vi "CreatePublicEvents.vi"(8 "error in (no error)":errorcluster, 11 "Control Experiment":refnum<class "SMO.Control Experiment.lvclass">) -> (0 "error out":errorcluster, 3 "Control Experiment out":refnum<class "SMO.Control Experiment.lvclass">)   [LabVIEW 2019, in "SMO.Control Experiment.lvclass"]
doc: "---------------------------------------------------------------\nJKI State Machine Objects™\nhttp://jki.net/state-machine-objects/\nCopyright (C) 2005-2015, JKI <info@jki.net>\nALL RIGHTS RESERVEDJKI State Machine Objects (SMO) 1.0.0.4\nJKI - JKI\nCopyright (c) 2015, JKI"
uses:
  SMO.Control Experiment.lvclass
  Typedefs/PublicEvents--Control Experiment.getUIconfig.ctl
  SMO.Control Experiment UI/Typedefs/UI Config--Cluster.ctl
  SMO.Control Experiment UI/Typedefs/UI Channels--Cluster.ctl
  SMO.Control Experiment UI/Typedefs/UI Channels.AI--Cluster.ctl
  SMO.Control Experiment UI/Typedefs/UI Channels.Device--Cluster.ctl
  Control Experiment/Typedefs/KH Mode-enum.ctl
  SMO.Control Experiment UI/Typedefs/UI Channels.KH--Cluster.ctl
  <userlib>/LevyLab/Krohn Hite 7008/typedefs/Input Configuration-Enum.ctl
  <userlib>/LevyLab/Krohn Hite 7008/typedefs/Gain-Enum.ctl
  <userlib>/LevyLab/Krohn Hite 7008/typedefs/Shunt-Enum.ctl
  SMO.Control Experiment UI/Typedefs/UI Channels.AO--Cluster.ctl
  Control Experiment/Typedefs/Instrument--enum.ctl
  <userlib>/LevyLab/Krohn Hite 7008/typedefs/Coupling-Enum.ctl
  <userlib>/LevyLab/Krohn Hite 7008/typedefs/Filter-Enum.ctl
  Typedefs/PublicEvents--Control Experiment.getKHShuntType.ctl
  SMO.Control Experiment.lvclass/SMO.Control Experiment.ctl
  <userlib>/LevyLab/Instrument Framework/SMOs/Instrument/Instrument.lvclass
  <userlib>/LevyLab/Krohn Hite 7008/Instrument.KH7008.lvclass
  Control Experiment/Control Experiment.lvclass
  SMO.Control Experiment UI/SMO.Control Experiment UI.lvclass
panel:
  # "For instructions on how to use the JKI State Machine Objects, examples and video tutorials, visit:\nhttp://jki.net/state-machine-objects/\n\nJKI State Machine Objects™\nhttp://jki.net/state-machine-objects/\nCopyright (C) 2005-2015, JKI <info@jki.net>\nALL RIGHTS RESERVED"
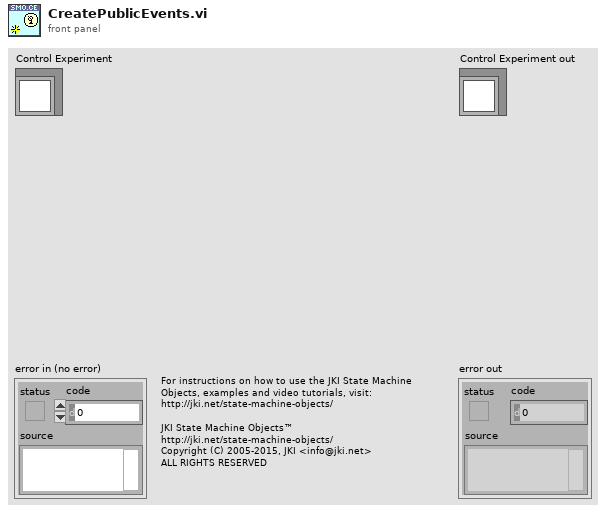
[diagram p1: front panel]
types:
  T1 = typedef "SMO.Control Experiment.lvclass/PublicEvents--Control Experiment.getKHShuntType.ctl" = enum16{"500", "10M"}
  T2 = typedef "SMO.Control Experiment.lvclass/PublicEvents--Control Experiment.getUIconfig.ctl" = cluster{"UI Configuration":T3}
  T3 = typedef "SMO.Control Experiment.lvclass/UI Config--Cluster.ctl" = cluster{"Metadata":cluster{"Sample (SAXXXX)":string, "Device (YYYYMMDD)":string, "Description":string, "Username":string, "Default Path":path}, "Number of AI":i32, "UI Channels []":T4[], "Instruments":cluster{"Lockin Address":string, "Krohn Hite?":bool, "KH Addresses":refnum<visa-resource-name>[], "Strain Cell?":bool, "Strain Cell Address":refnum<visa-resource-name>, "C Bridge?":bool, "Capacitance Bridge Address":refnum<visa-resource-name>, "Instrument":T13}, "Krohn Hite":cluster{"Defualt Shunt Resistor":T11, "Default Gain":T10, "Coupling":T14, "Bandwidth Filter":T15}}
  T4 = typedef "SMO.Control Experiment UI.lvclass/UI Channels--Cluster.ctl" = cluster{"AI":T5, "Device":T6, "KH":T8, "AO":T12}
  T5 = typedef "SMO.Control Experiment UI.lvclass/UI Channels.AI--Cluster.ctl" = cluster{"Channel":u32, "Gain":dbl}
  T6 = typedef "SMO.Control Experiment UI.lvclass/UI Channels.Device--Cluster.ctl" = cluster{"Electrode":string, "Configuration":T7, "Label":u16}
  T7 = typedef "Control Experiment.lvclass/KH Mode-enum.ctl" = enum16{"Ground", "Current", "Voltage (SE)", "Voltage (Diff)", "Gate"}
  T8 = typedef "SMO.Control Experiment UI.lvclass/UI Channels.KH--Cluster.ctl" = cluster{"Channel":u16, "Configuration":T9, "Gain":T10, "Shunt Resistor":T11}
  T9 = typedef "Instrument.KH7008.lvclass/Input Configuration-Enum.ctl" = enum16{"Ground", "SE+ (-gnd)", "SE- (+gnd)", "Differential"}
  T10 = typedef "Instrument.KH7008.lvclass/Gain-Enum.ctl" = enum16{"1x", "10x", "100x", "1000x"}
  T11 = typedef "Instrument.KH7008.lvclass/Shunt-Enum.ctl" = enum16{"Open", "50 Ohms", "500 Ohms", "5k Ohms", "50k Ohms", "10M Ohm"}
  T12 = typedef "SMO.Control Experiment UI.lvclass/UI Channels.AO--Cluster.ctl" = cluster{"Channel":u32, "Gain":dbl}
  T13 = typedef "Control Experiment.lvclass/Instrument--enum.ctl" = enum16{"----- AFM/EBL -----", "AGILENT", "CYPHER", "Gemini2", "JEOL", "MFP3D", "----- Cryostat -----", "CF900", "DR200", "MNK", "PPMS (simulated)", "PPMS 1", "PPMS 2", "PPMS 3", "----- Optics -----", "THz 1 (Element 2/Montana)", "THz 2 (Tsunami/Janis)"}
  T14 = typedef "Instrument.KH7008.lvclass/Coupling-Enum.ctl" = enum16{"AC", "DC"}
  T15 = typedef "Instrument.KH7008.lvclass/Filter-Enum.ctl" = enum16{"OFF", "ON"}
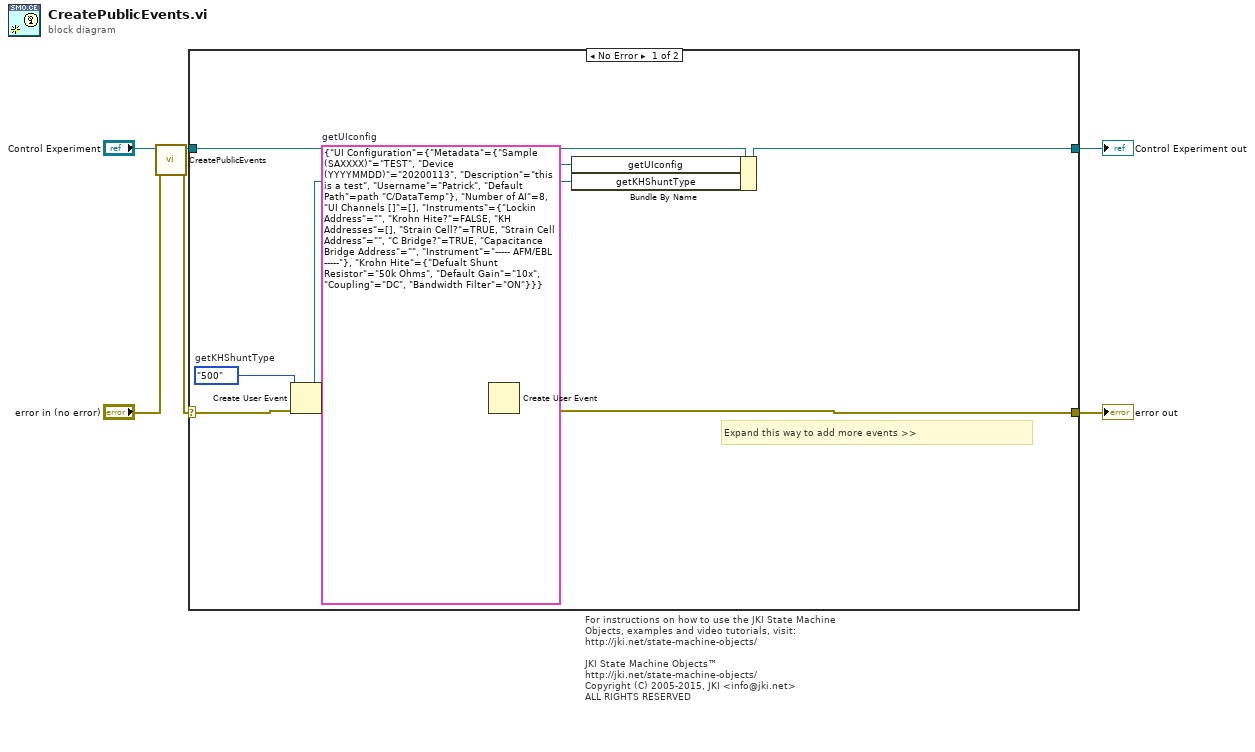
[diagram p0: block diagram]
diagram:
  # "For instructions on how to use the JKI State Machine Objects, examples and video tutorials, visit:\nhttp://jki.net/state-machine-objects/\n\nJKI State Machine Objects™\nhttp://jki.net/state-machine-objects/\nCopyright (C) 2005-2015, JKI <info@jki.net>\nALL RIGHTS RESERVED"
  n1 = call-parent "CreatePublicEvents.vi"("error in (no error)"="error in (no error)", "Instrument"="Control Experiment") -> ("error out"=w1:errorcluster, "Instrument out"=w3:refnum<class "SMO.Control Experiment.lvclass">)  [unwired: 8 in]
  n2 = case shown="No Error" w1 {
    selector: w1 -> [w14 w17]
    tunnel: [w12 w17] -> w5
    tunnel: [w13 w16] -> w6
    tunnel: w3 -> [w15 w16]
    frame No Error {
      w8 = PublicEvents--Control_Experiment.getKHShuntType."500"  # getKHShuntType
      w11 = T2 {"UI Configuration"={"Metadata"={"Sample (SAXXXX)"="TEST", "Device (YYYYMMDD)"="20200113", "Description"="this is a test", "Username"="Patrick", "Default Path"=path "C:/DataTemp"}, "Number of AI"=8, "UI Channels []"=[], "Instruments"={"Lockin Address"="", "Krohn Hite?"=FALSE, "KH Addresses"=[], "Strain Cell?"=TRUE, "Strain Cell Address"="", "C Bridge?"=TRUE, "Capacitance Bridge Address"="", "Instrument"=enum."----- AFM/EBL -----"}, "Krohn Hite"={"Defualt Shunt Resistor"=enum."50k Ohms", "Default Gain"=enum."10x", "Coupling"=enum."DC", "Bandwidth Filter"=enum."ON"}}}  # getUIconfig
      # "Expand this way to add more events >>"
      n3 = Create User Event(user event datatype=w8, error in=w14) -> (user event=w7:refnum<user-event>, error out=w9:errorcluster)
      n4 = Create User Event(user event datatype=w11, error in=w9) -> (user event=w10:refnum<user-event>, error out=w12:errorcluster)
      n5 = Bundle By Name(cluster=w15, "getUIconfig"=w10, "getKHShuntType"=w7) -> (w13:refnum<class "SMO.Control Experiment.lvclass">)
    }
    frame Error {
    }
  }
  "error out" <- w5
  "Control Experiment out" <- w6
